vi "Init Core.vi"(0 "Display State In":T3={"Events"={"Navigation Complete Event"=refnum, "Source Changed Event"=refnum, "Document Title Changed Event"=refnum, "Status Bar Text Changed"=refnum, "Web Message Received"=refnum, "Window Close Requested"=refnum, "DOM Loaded"=refnum, "Navigation Started Event"=refnum}, "Paths"={"Webview2 Native"=path "C:/Users/kleins/Desktop/webview2/microsoft.web.webview2.1.0.1370.28/build/native", "Edge Application"=path "", "User Data"=path ""}, "Environment Options"={"additionalBrowserArguments"="", "language"="", "targetCompatibleBrowserVersion"="", "allowSingleSignOnUsingOSPrimaryAccount"=FALSE}, "Res"=refnum}, 5 "Path Overrides":T2, 7 "Environment Options":T1, 9 "Container State":T5, 11 "error in (no error)":errorcluster) -> (4 "Display State Out":T3={"Events"={"Navigation Complete Event"=refnum, "Source Changed Event"=refnum, "Document Title Changed Event"=refnum, "Status Bar Text Changed"=refnum, "Web Message Received"=refnum, "Window Close Requested"=refnum, "DOM Loaded"=refnum, "Navigation Started Event"=refnum}, "Paths"={"Webview2 Native"=path "C:/Users/kleins/Desktop/webview2/microsoft.web.webview2.1.0.1370.28/build/native", "Edge Application"=path "", "User Data"=path ""}, "Environment Options"={"additionalBrowserArguments"="", "language"="", "targetCompatibleBrowserVersion"="", "allowSingleSignOnUsingOSPrimaryAccount"=FALSE}, "Res"=refnum}, 15 "error out":errorcluster)   [LabVIEW 2020, in "WebView2 Control.xctl"]
uses:
  WebView2 Control.xctl
  <vilib>/_xctls/Container State.ctl
  State.ctl
  Events.ctl
  Navigation Event Data.ctl
  Source Changed Event Data.ctl
  Navigation Start Event Data.ctl
  E:/Labview/LV 2020/Libs/WebView2/LV-WebView2/Source/Libs/Microsoft.Web.WebView2.Core.dll
  Libs/Microsoft.Web.WebView2.Core.dll
  Paths.ctl
  Core Env Options.ctl
  Res.ctl
  E:/Labview/LV 2020/Libs/WebView2/LV-WebView2/Source/Libs/Microsoft.Web.WebView2.WinForms.dll
  Libs/Microsoft.Web.WebView2.WinForms.dll
  <vilib>/_xctls/XControlSupport.lvlib
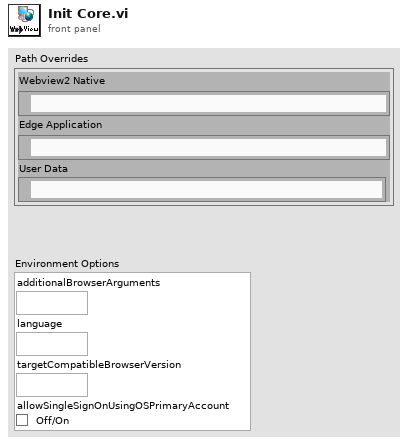
[diagram p1: front panel]
types:
  T1 = typedef "WebView2 Control.xctl/Core Env Options.ctl" = cluster{"additionalBrowserArguments":string, "language":string, "targetCompatibleBrowserVersion":string, "allowSingleSignOnUsingOSPrimaryAccount":bool}
  T2 = typedef "WebView2 Control.xctl/Paths.ctl" = cluster{"Webview2 Native":path, "Edge Application":path, "User Data":path}
  T3 = typedef "WebView2 Control.xctl/State.ctl" = cluster{"Events":T4, "Paths":T2, "Environment Options":T1, "Res":refnum<data-value>}
  T4 = typedef "WebView2 Control.xctl/Events.ctl" = cluster{"Navigation Complete Event":refnum<user-event>, "Source Changed Event":refnum<user-event>, "Document Title Changed Event":refnum<user-event>, "Status Bar Text Changed":refnum<user-event>, "Web Message Received":refnum<user-event>, "Window Close Requested":refnum<user-event>, "DOM Loaded":refnum<user-event>, "Navigation Started Event":refnum<user-event>}
  T5 = typedef "XControlSupport.lvlib/Container State.ctl" = cluster{"Indicator?":bool, "Run Mode?":bool, " Refnum":refnum<vi>}
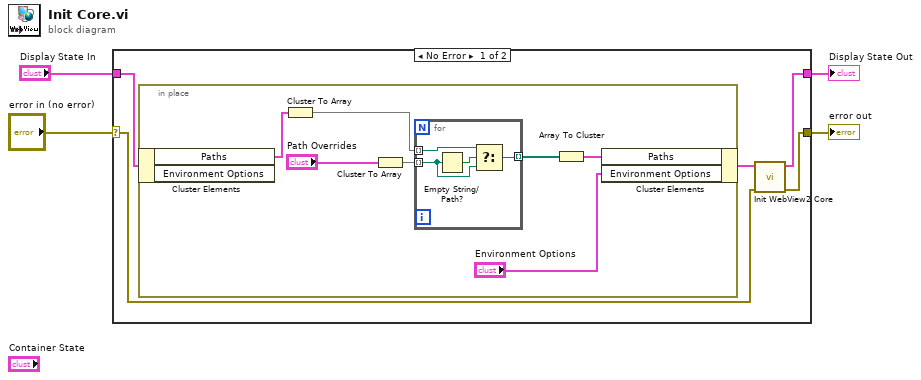
[diagram p0: block diagram]
diagram:
  n1 = case shown="No Error" "error in (no error)" {
    selector: "error in (no error)" -> [w7 w22]
    tunnel: [w9 w22] -> w3
    tunnel: [w6 w21] -> w2
    tunnel: "Display State In" -> [w5 w21]
    frame No Error {
      n2 = in-place {
        n3 = in-place-cluster #1(w5) -> ("Paths"=w16:T2)  [unwired: 1 out]
        n4 = Cluster To Array(cluster=w16) -> (array=w15:path[])
        n5 = Cluster To Array(cluster="Path Overrides") -> (array=w12:path[])
        n6 = for {
          tunnel: [w20] -> w14 mode=indexing
          tunnel: w15 -> [w17] mode=indexing
          tunnel: w12 -> [w18] mode=indexing
          n7 = Empty String/Path?(string/path=w18) -> (empty?=w19:bool)
          n8 = Select(t=w17, s=w19, f=w18) -> (s? t:f=w20:path)
        }
        n9 = Array To Cluster(array=w14) -> (cluster=w13:cluster{"[0]":path, "[1]":path, "[2]":path})
        n10 = in-place-cluster #1("Paths"=w13, "Environment Options"="Environment Options") -> (w8:T3)
      }
      n11 = call "Init WebView2 Core.vi"("error in (no error)"=w7, "Display State In"=w8) -> ("error out"=w9:errorcluster, "Display State In 2"=w6:T3)  [unwired: 8 in]
    }
    frame Error {
    }
  }
  "Display State Out" <- w2
  "error out" <- w3
